vi "Write VISA resource.vi"(8 "error in (no error)":errorcluster, 10 "VISA resource":refnum<visa-resource-name>, 11 "VISA Instrument in":refnum<class "VISA Instrument.lvclass">) -> (0 "error out":errorcluster, 3 "VISA Instrument out":refnum<class "VISA Instrument.lvclass">)   [LabVIEW 2015, in "VISA Instrument.lvclass"]
uses:
  VISA Instrument.lvclass
  VISA Instrument.lvclass/VISA Instrument.ctl
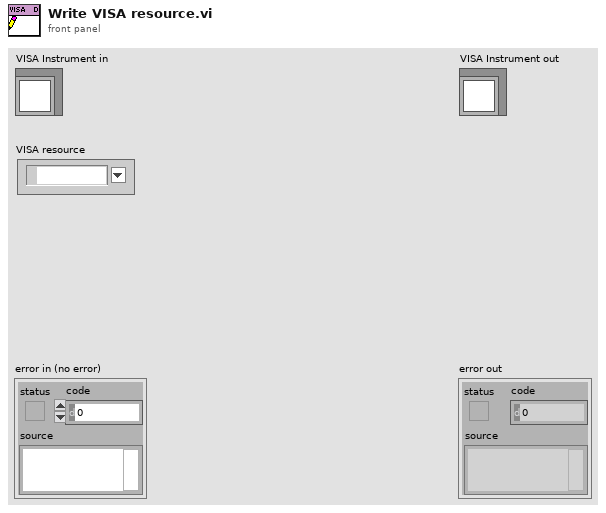
[diagram p1: front panel]
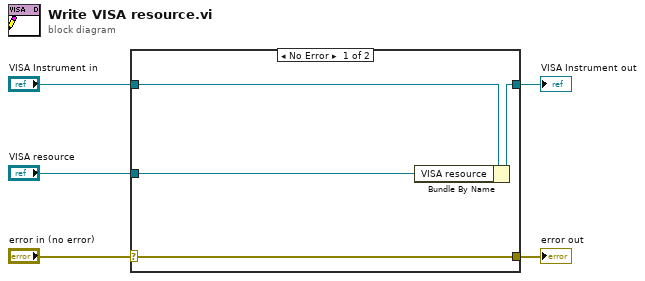
[diagram p0: block diagram]
diagram:
  n1 = case shown="No Error" "error in (no error)" {
    selector: "error in (no error)" -> [w9 w10]
    tunnel: [w9 w10] -> w4
    tunnel: [w7 w11] -> w2
    tunnel: "VISA Instrument in" -> [w8 w11]
    tunnel: "VISA resource" -> [w6 _]
    frame No Error {
      n2 = Bundle By Name(cluster=w8, "VISA resource"=w6) -> (w7:refnum<class "VISA Instrument.lvclass">)
    }
    frame Error {
    }
  }
  "error out" <- w4
  "VISA Instrument out" <- w2
